vi "多设备同步_外部时钟源.vi"() -> ()   [LabVIEW 2013]
uses:
  <userlib>/ArtDAQ/_SubVI/ArtDAQ_CreateAIVoltageChan.vi
  <userlib>/ArtDAQ/_SubVI/ArtDAQ_CfgSampClkTiming.vi
  <userlib>/ArtDAQ/_SubVI/ArtDAQ_Read Analog DBL NChan NSamp.vi
panel:
  in  "采集卡类型选择":enum16{"同步卡", "异步卡"}(ring)
  in  "时钟源0":string(combo)="/Dev1/PFI2"
  in  "时钟源1":string(combo)="/Dev2/PFI2"
  in  "通道1":string(combo)="Dev2/ai0"
  in  "通道0":string(combo)="Dev1/ai0"
  out "ErrorOutput":errorcluster caption="错误输出"
  out "?":dbl[][](graph)
  out "?":dbl[][](graph)
  in  "停止":bool
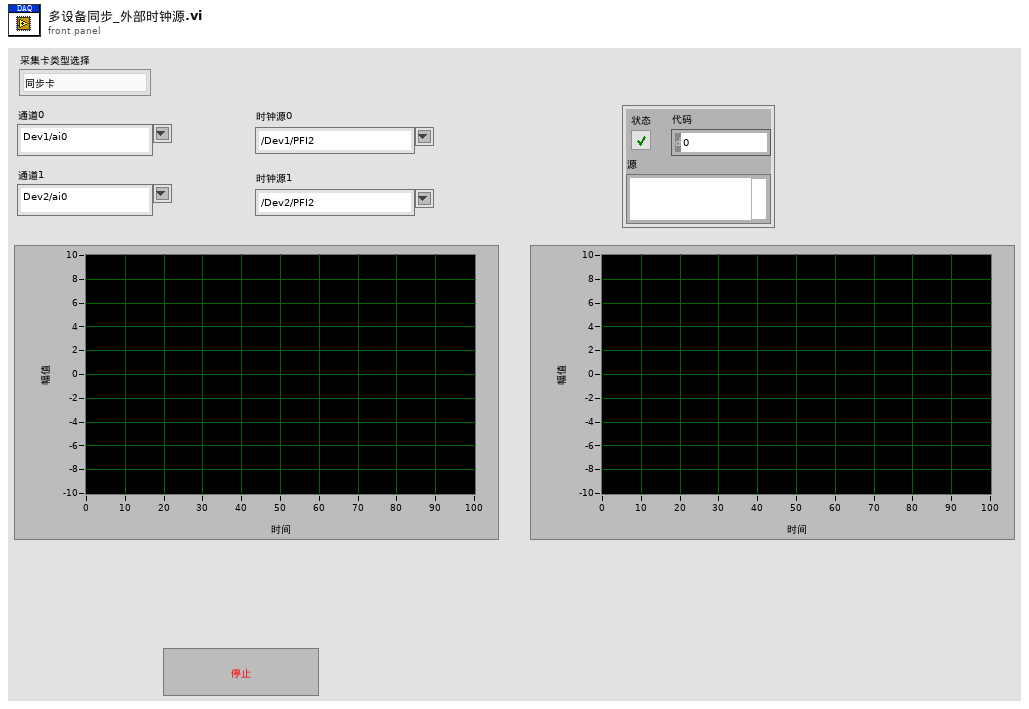
[diagram p1: front panel]
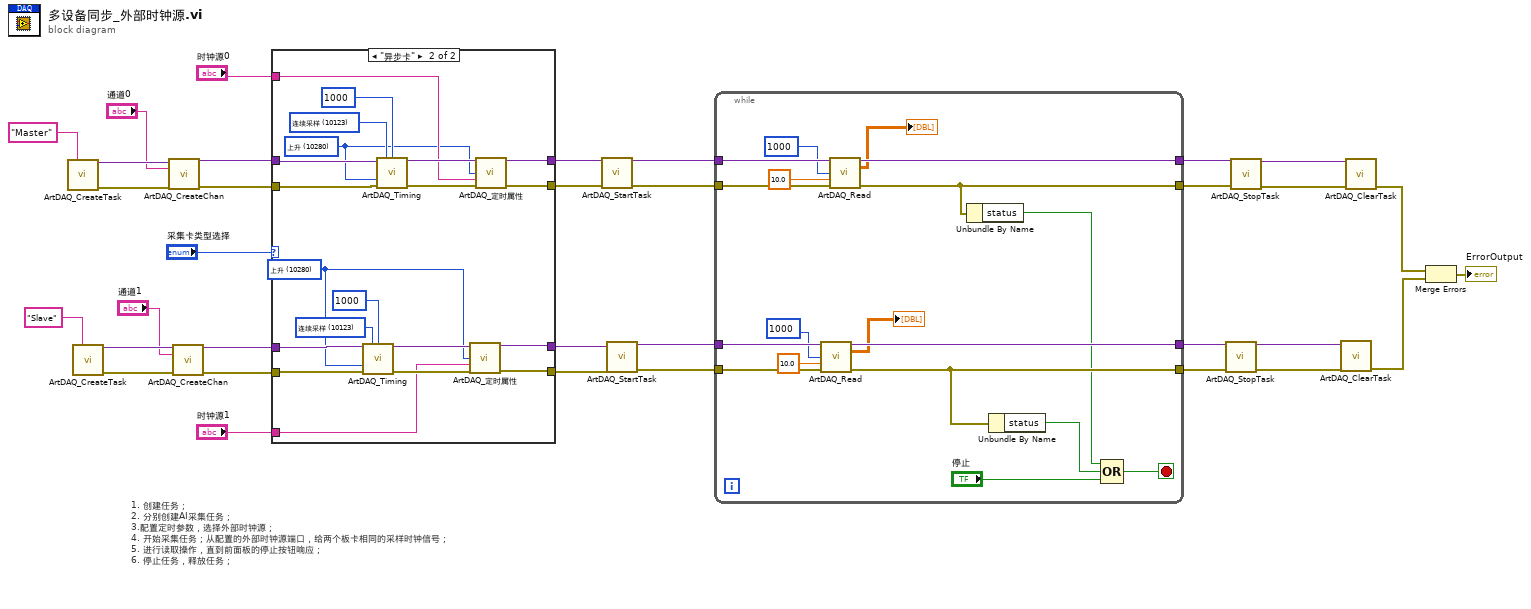
[diagram p0: block diagram]
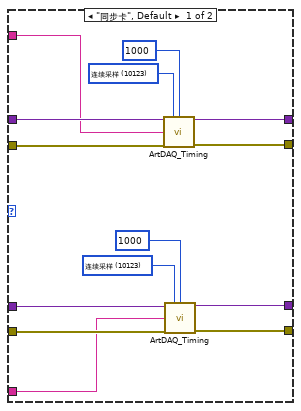
[diagram p2: hidden frame]
diagram:
  # "1. 创建任务；\n2. 分别创建AI采集任务；\n3.配置定时参数，选择外部时钟源；\n4. 开始采集任务；从配置的外部时钟源端口，给两个板卡相同的采样时钟信号；\n5. 进行读取操作，直到前面板的停止按钮响应；\n6. 停止任务，释放任务；"
  n1 = call <userlib>:"ArtDAQ_CreateTask.vi"("任务名称"="Master" ("TaskName")) -> ("任务句柄"=w34:variant, "错误输出"=w33:errorcluster)  [unwired: 13 in]
  n2 = call <userlib>:"ArtDAQ_CreateTask.vi"("任务名称"="Slave" ("TaskName")) -> ("任务句柄"=w32:variant, "错误输出"=w31:errorcluster)  [unwired: 13 in]
  n3 = call-poly <userlib>:"ArtDAQ_CreateChan.vi"("任务句柄"=w34, "物理通道"="通道0", "错误输入"=w33) -> ("任务句柄"=w27:variant, "错误输出"=w28:errorcluster)  [unwired: 11 in]
  n4 = call-poly <userlib>:"ArtDAQ_CreateChan.vi"("任务句柄"=w32, "物理通道"="通道1", "错误输入"=w31) -> ("任务句柄"=w30:variant, "错误输出"=w29:errorcluster)  [unwired: 11 in]
  n5 = case shown="\"异步卡\"" "采集卡类型选择" {
    tunnel: w30 -> [w48 w56]
    tunnel: w29 -> [w47 w55]
    tunnel: w28 -> [w46 w63]
    tunnel: w27 -> [w45 w64]
    tunnel: [w44 w53] -> w26
    tunnel: [w43 w51] -> w25
    tunnel: [w42 w61] -> w24
    tunnel: [w41 w59] -> w23
    tunnel: "时钟源0" -> [w38 w58]
    tunnel: "时钟源1" -> [w37 w49]
    frame "同步卡", Default {
      w39 = 10123 items=["有限点采样"=10178, "连续采样"=10123] ("采样模式")
      w40 = 10123 items=["有限点采样"=10178, "连续采样"=10123] ("采样模式")
      n6 = call-poly <userlib>:"ArtDAQ_Timing.vi"("任务句柄"=w45, "采样模式"=w40, "每通道采样数"=1000, "源"=w38, "错误输入"=w46) -> ("任务句柄"=w42:variant, "错误输出"=w41:errorcluster)  [unwired: 9 in]
      n7 = call-poly <userlib>:"ArtDAQ_Timing.vi"("任务句柄"=w48, "采样模式"=w39, "每通道采样数"=1000, "源"=w37, "错误输入"=w47) -> ("任务句柄"=w44:variant, "错误输出"=w43:errorcluster)  [unwired: 9 in]
    }
    frame "异步卡" {
      w50 = 10280 items=["上升"=10280, "下降"=10171] ("边沿")
      w57 = 10280 items=["上升"=10280, "下降"=10171] ("边沿")
      w67 = 10123 items=["有限点采样"=10178, "连续采样"=10123] ("采样模式")
      w68 = 10123 items=["有限点采样"=10178, "连续采样"=10123] ("采样模式")
      n8 = call-poly <userlib>:"ArtDAQ_Timing.vi"("任务句柄"=w56, "采样模式"=w67, "每通道采样数"=1000, "有效边沿"=w50, "错误输入"=w55) -> ("任务句柄"=w54:variant, "错误输出"=w52:errorcluster)  [unwired: 9 in]
      n9 = call-poly <userlib>:"ArtDAQ_Timing.vi"("任务句柄"=w64, "采样模式"=w68, "每通道采样数"=1000, "有效边沿"=w57, "错误输入"=w63) -> ("任务句柄"=w62:variant, "错误输出"=w60:errorcluster)  [unwired: 9 in]
      n10 = call-poly "ArtDAQ_定时属性.vi"("任务句柄"=w54, "边沿"=w50, "转换时钟源"=w49, "错误输入"=w52) -> ("任务句柄"=w53:variant, "错误输出"=w51:errorcluster)  [unwired: 10 in]
      n11 = call-poly "ArtDAQ_定时属性.vi"("任务句柄"=w62, "边沿"=w57, "转换时钟源"=w58, "错误输入"=w60) -> ("任务句柄"=w61:variant, "错误输出"=w59:errorcluster)  [unwired: 10 in]
    }
  }
  n12 = call <userlib>:"ArtDAQ_StartTask.vi"("任务句柄"=w24, "错误输入"=w23) -> ("任务句柄"=w22:variant, "错误输出"=w21:errorcluster)  [unwired: 12 in]
  n13 = call <userlib>:"ArtDAQ_StartTask.vi"("任务句柄"=w26, "错误输入"=w25) -> ("任务句柄"=w20:variant, "错误输出"=w19:errorcluster)  [unwired: 12 in]
  n14 = while {
    tunnel: w22 -> [w86]
    tunnel: w21 -> [w85]
    tunnel: w20 -> [w84]
    tunnel: w19 -> [w83]
    tunnel: [w82] -> w16
    tunnel: [w73] -> w15
    tunnel: [w81] -> w12
    tunnel: [w72] -> w11
    stop <- w78 stop-if-true
    n15 = call-poly <userlib>:"ArtDAQ_Read.vi"("任务句柄"=w84, "每通道采样数"=1000 ("NumSampsPerChan"), "超时s"=10.0 ("Timeout"), "错误输入"=w83) -> ("任务句柄"=w81:variant, "数据"=→"?":dbl[][], "错误输出"=w72:errorcluster)  [unwired: 7 in, 2 out]
    n16 = call-poly <userlib>:"ArtDAQ_Read.vi"("任务句柄"=w86, "每通道采样数"=1000 ("NumSampsPerChan"), "超时s"=10.0 ("Timeout"), "错误输入"=w85) -> ("任务句柄"=w82:variant, "数据"=→"?":dbl[][], "错误输出"=w73:errorcluster)  [unwired: 7 in, 2 out]
    n17 = Unbundle By Name(w73) -> ("status"=w71:bool)
    n18 = Unbundle By Name(w72) -> ("status"=w80:bool)
    n19 = Compound Arithmetic op=OR(w71, w80, "停止") -> (w78:bool)
  }
  n20 = call <userlib>:"ArtDAQ_StopTask.vi"("任务句柄"=w12, "错误输入"=w11) -> ("任务句柄"=w13:variant, "错误输出"=w14:errorcluster)  [unwired: 12 in]
  n21 = call <userlib>:"ArtDAQ_StopTask.vi"("任务句柄"=w16, "错误输入"=w15) -> ("任务句柄"=w18:variant, "错误输出"=w17:errorcluster)  [unwired: 12 in]
  n22 = call <userlib>:"ArtDAQ_ClearTask.vi"("任务句柄"=w13, "错误输入"=w14) -> ("错误输出"=w9:errorcluster)  [unwired: 13 in]
  n23 = call <userlib>:"ArtDAQ_ClearTask.vi"("任务句柄"=w18, "错误输入"=w17) -> ("错误输出"=w10:errorcluster)  [unwired: 13 in]
  n24 = Merge Errors(w10, w9) -> (→"ErrorOutput":errorcluster)
